vi "Get Handler by Name.vi"(8 "error in":errorcluster, 11 "Name":string) -> (0 "error out":errorcluster, 3 "Handler out":refnum<class "Handler.lvclass">)   [LabVIEW 2024, in "hse-logger.lvlib"]
doc: "Returns a Handler from the logger specified by name.\nIf name was not found, returns a basis handler without functionality and raise an error \"510802 - Handler name not found\".\n\n____\nHAMPEL SOFTWARE ENGINEERING v2.2.2 (2025-01-16 15:41)"
uses:
  <vilib>/Hampel Software Engineering/HSE Logger/hse-logger.lvlib
  <vilib>/Hampel Software Engineering/HSE Logger/Handler/Handler.lvclass
  <vilib>/Hampel Software Engineering/HSE Logger/FGV Actions.ctl
  <vilib>/Hampel Software Engineering/HSE Logger/Logger/Logger.lvclass
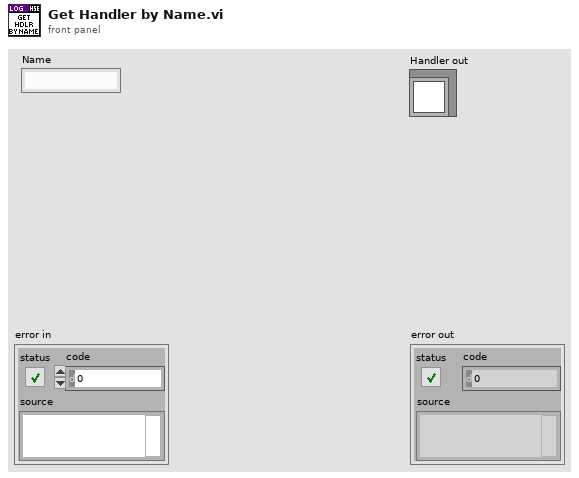
[diagram p1: front panel]
types:
  T1 = typedef "hse-logger.lvlib/FGV Actions.ctl" = enum16{"Set", "Get"}
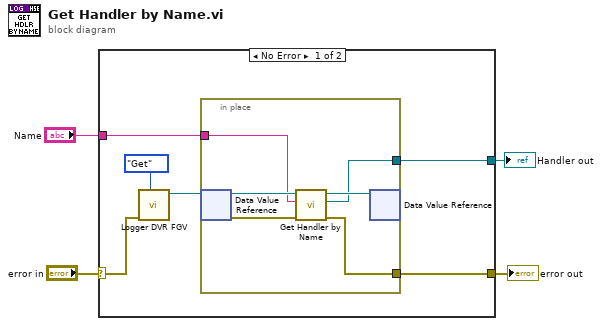
[diagram p0: block diagram]
diagram:
  n1 = case shown="No Error" "error in" {
    selector: "error in" -> [w10 w17]
    tunnel: [w6 w17] -> w3
    tunnel: "Name" -> [w8 _]
    tunnel: [w7 _] -> w1
    frame No Error {
      n2 = call <vilib>:"Logger DVR FGV.vi"("FGV Actions"=FGV_Actions."Get", "error in"=w10) -> ("Logger DVR"=w9:refnum<data-value>)  [unwired: 8 in, 1 out]
      n3 = in-place {
        in-place-border: w8 -> [w15]
        in-place-border: [w13] -> w7
        in-place-border: [w12] -> w6
        n4 = in-place-dvr #1(w9) -> (w16:refnum<class "Logger.lvclass">, w11:errorcluster)
        n5 = call-dynamic "Get Handler by Name.vi"("error in"=w11, "Name"=w15, "Logger in"=w16) -> ("error out"=w12:errorcluster, "Handler out"=w13:refnum<class "Handler.lvclass">, "Logger out"=w14:refnum<class "Logger.lvclass">)  [unwired: 6 in]
        n6 = in-place-dvr #1(w14) -> ()  [unwired: 2 out]
      }
    }
    frame Error {
    }
  }
  "error out" <- w3
  "Handler out" <- w1
